vi "Execute_Row.vi"(3 "Simulate/Run":T2, 5 "Traverse line":T3 {"Row Duration (mins)" format="%#.1f"; "Row No" min=0; "Trace Gas Concentration (%)" min=0.0 format="%#.2f"; "Emission Rate (l/min)" format="%#.2f"; "Tunnel Speed" format="%#.2f"; "Start X" format="%#.2f"; "Start Y" format="%#.2f"; "Start Z" format="%#.2f"; "End X" format="%#.2f"; "End Y" format="%#.2f"; "End Z" format="%#.2f"; "Averaging time (min)" min=0.0 format="%#.2f"}) -> (1 "Status":T1, 2 "Traverse line out":T3 {"Row Duration (mins)" format="%#.1f"; "Row No" min=0; "Trace Gas Concentration (%)" min=0.0 format="%#.2f"; "Emission Rate (l/min)" format="%#.2f"; "Tunnel Speed" format="%#.2f"; "Start X" format="%#.2f"; "Start Y" format="%#.2f"; "Start Z" format="%#.2f"; "End X" format="%#.2f"; "End Y" format="%#.2f"; "End Z" format="%#.2f"; "Averaging time (min)" min=0.0 format="%#.2f"})   [LabVIEW 2014]
uses:
  Traverse_cluster.ctl
  Spacing.ctl
  Controls/Multi_run_mode.ctl
  Controls/User_Specific_mode.ctl
  Multi_Run_Status.ctl
  Controls/Setup.ctl
  Controls/Save_Data.ctl
  Globals/Constants_global.vi
  Globals/Extra_Commands_Global.vi
  Globals/Trav_pos_global.vi
panel:
  # "X           Y            Z"
  # "Start"
  # "End"
  # "X           Y            Z"
  # "Start"
  # "End"
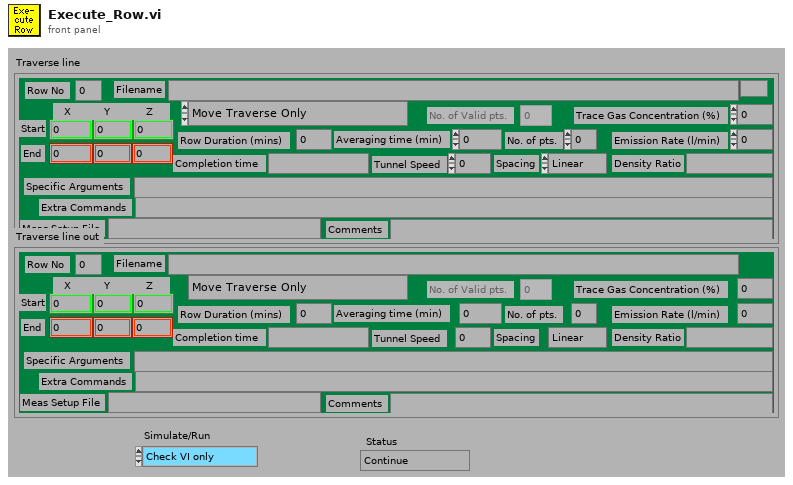
[diagram p1: front panel]
types:
  T1 = typedef "Multi_Run_Status.ctl" = enum16{"Continue", "Jump to Next Point", "Jump to Next Row", "Jump To Fall Back", "Terminate Run"}
  T2 = typedef "User_Specific_mode.ctl" = enum16{"Check VI only", "Run VI"}
  T3 = typedef "Traverse_cluster.ctl" = cluster{"Start X":dbl, "Start Y":dbl, "Start Z":dbl, "End X":dbl, "End Y":dbl, "End Z":dbl, "No. of pts.":i32, "Spacing":T4, "Filename":path, "Tunnel Speed":dbl, "Averaging time (min)":dbl, "Extra Commands":string, "Specific Arguments":string, "Emission Rate (l/min)":dbl, "Trace Gas Concentration (%)":dbl, "Density Ratio":string, "Comments":string, "Row No":i32, "Row Type Selector":T5, "Completion time":string, "Row Duration (mins)":dbl, "No. of Valid pts.":i32, "Meas Setup File":string}
  T4 = typedef "Spacing.ctl" = enum16{"Linear", "Log", "Gauss", "Specified", "N/A"}
  T5 = typedef "Multi_run_mode.ctl" = enum16{"Move Traverse Only", "Set Tunnel Speed Only", "Set Source Only", "Set Measurement Conditions", "Single Measurement", "Vertical Profile", "Lateral Profile", "Longitudinal Profile", "Explore Volume", "Multi-Axis Profile", "Auto Calibrate", "Meas Fast FID Bkgnd", "Check Beam Power", "Scanning Valve Measurement", "Run VI Named:", "Set ADAM Ch", "Wait (minutes)", "Send Message", "Synchronize With:", "Fall Back to this Row", "Turn Off Row Repeating", "Blank Row", "Traverse 3D Volume"}
  T6 = typedef "Save_Data.ctl" = enum16{"Save No Data", "Save Data"}
  T7 = typedef "Setup.ctl" = enum16{"Run Program", "Show Setup", "Save Current Setup", "Setup Front Panel"}
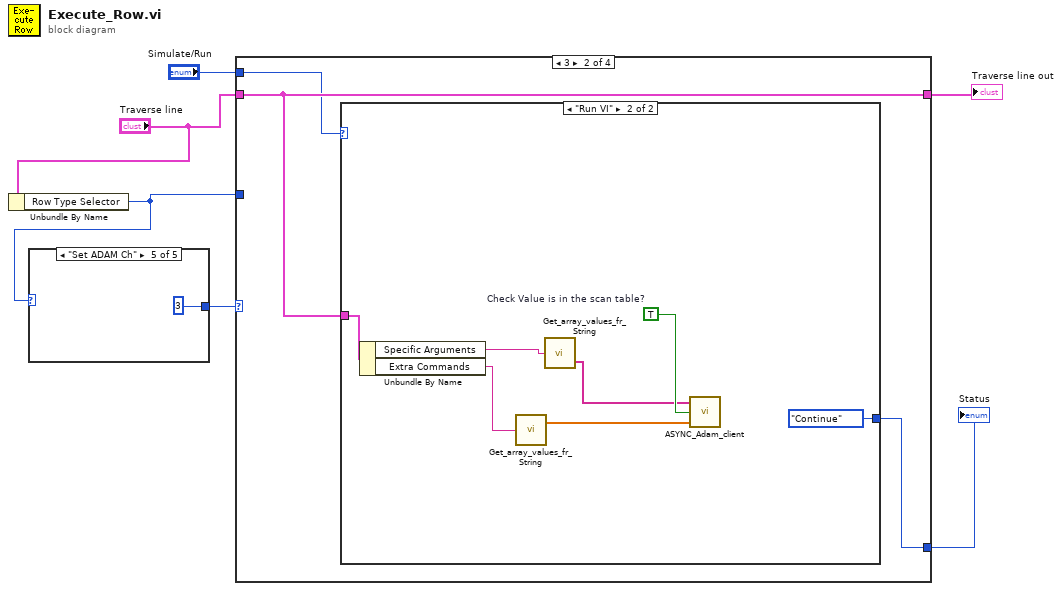
[diagram p0: block diagram]
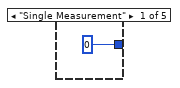
[diagram p2: hidden frame]
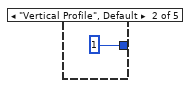
[diagram p3: hidden frame]
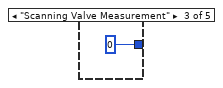
[diagram p4: hidden frame]
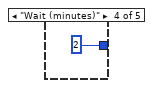
[diagram p5: hidden frame]
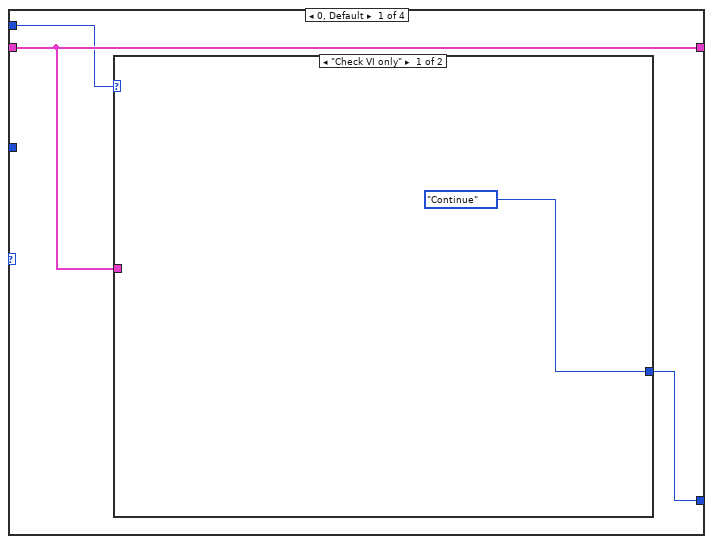
[diagram p6: hidden frame]
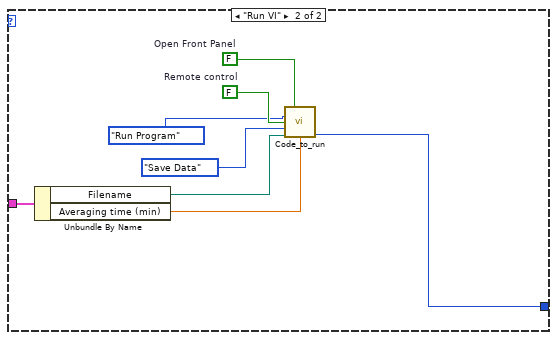
[diagram p7: hidden frame]
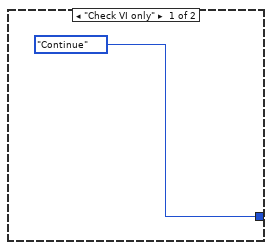
[diagram p8: hidden frame]
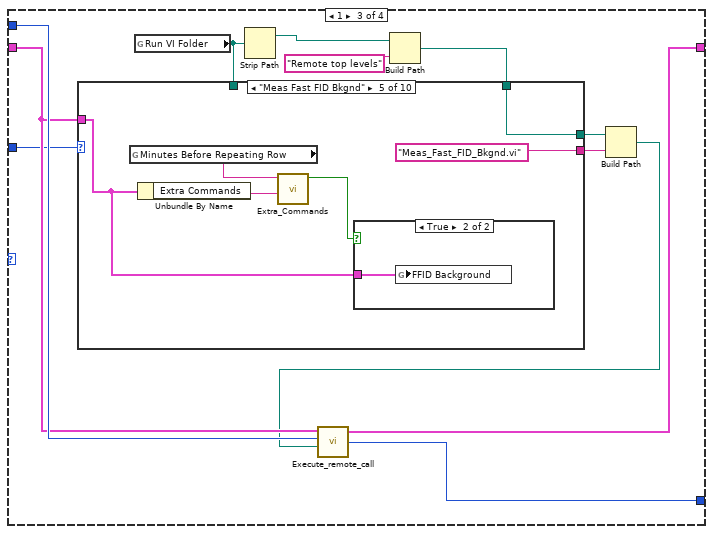
[diagram p9: hidden frame]
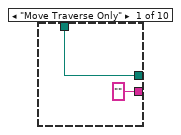
[diagram p10: hidden frame]
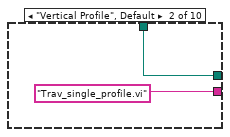
[diagram p11: hidden frame]
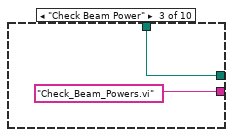
[diagram p12: hidden frame]
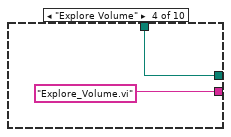
[diagram p13: hidden frame]
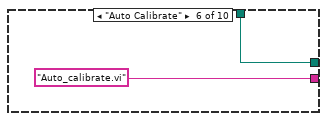
[diagram p15: hidden frame]
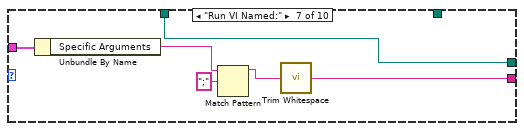
[diagram p16: hidden frame]
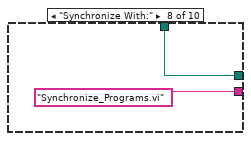
[diagram p17: hidden frame]
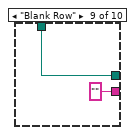
[diagram p18: hidden frame]
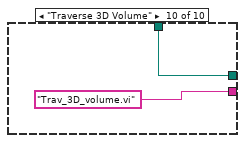
[diagram p19: hidden frame]
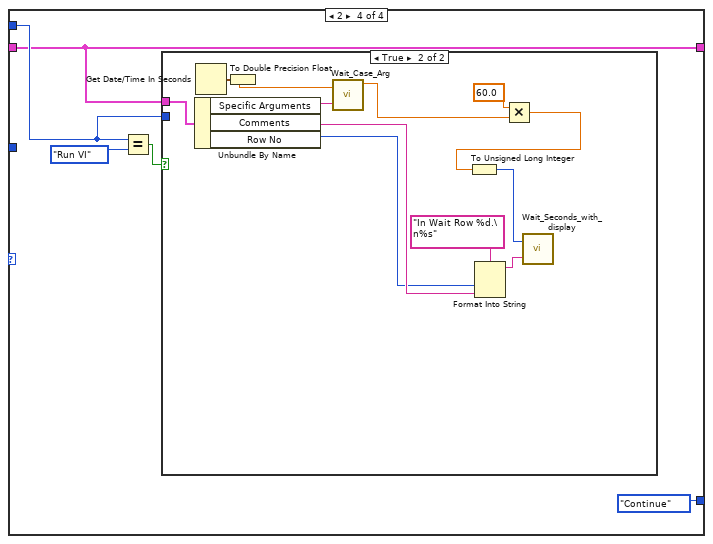
[diagram p20: hidden frame]
diagram:
  n1 = Unbundle By Name("Traverse line") -> ("Row Type Selector"=w2:T5)
  n2 = case shown="\"Set ADAM Ch\"" w2 {
    tunnel: [0 1 0 2 3] -> w3
    frame "Single Measurement" {
    }
    frame "Vertical Profile", Default {
    }
    frame "Scanning Valve Measurement" {
    }
    frame "Wait (minutes)" {
    }
    frame "Set ADAM Ch" {
    }
  }
  n3 = case shown="3" w3 {
    tunnel: [w14 w26 w42 Multi_Run_Status."Continue" ("Status")] -> w1
    tunnel: "Traverse line" -> [w13 w25 w44 w77]
    tunnel: [w13 w25 w46 w77] -> w6
    tunnel: "Simulate/Run" -> [w12 w24 w45 w79]
    tunnel: w2 -> [_ _ w43 _]
    frame 0, Default {
      n4 = case shown="\"Check VI only\"" w12 {
        tunnel: [Multi_Run_Status."Continue" ("Status") w23] -> w14
        tunnel: w13 -> [_ w22]
        frame "Check VI only" {
        }
        frame "Run VI" {
          w18 = FALSE  # Open Front Panel
          w20 = FALSE  # Remote control
          n5 = Unbundle By Name(w22) -> ("Filename"=w21:path, "Averaging time (min)"=w19:dbl)
          n6 = call "Code_to_run.vi"("Open Front Panel"=w18, "setup"=Setup."Run Program", "Remote control"=w20, "File"=Save_Data."Save Data", "Results Filename"=w21, "Averaging time (min)"=w19) -> ("Status"=w23:T1)  [unwired: 5 in, 4 out]
        }
      }
    }
    frame 3 {
      n7 = case shown="\"Run VI\"" w24 {
        tunnel: [Multi_Run_Status."Continue" ("Status") Multi_Run_Status."Continue" ("Status")] -> w26
        tunnel: w25 -> [_ w34]
        frame "Check VI only" {
        }
        frame "Run VI" {
          w32 = TRUE  # Check Value is in the scan table?
          n8 = Unbundle By Name(w34) -> ("Specific Arguments"=w31:string, "Extra Commands"=w29:string)
          n9 = call "Get_array_values_fr_String.vi"("String Value"=w29) -> ("Numeric Array"=w28:dbl[])  [unwired: 1 out]
          n10 = call "Get_array_values_fr_String.vi"("String Value"=w31) -> ("String array"=w30:string[])  [unwired: 1 out]
          n11 = call "ASYNC_Adam_client.vi"("Values"=w28, "Check Value is in the scan table?"=w32, "Channel Names"=w30) -> ()  [unwired: 2 out]
        }
      }
    }
    frame 1 {
      n12 = global read "Constants_global.vi" "Run VI Folder"() -> (w35:path)
      n13 = Strip Path(path=w35) -> (stripped path=w36:path)  [unwired: 1 out]
      n14 = Build Path(base path=w36, name or relative path="Remote top levels") -> (appended path=w40:path)
      n15 = case shown="\"Meas Fast FID Bkgnd\"" w43 {
        tunnel: w40 -> [w48 w50 w52 w54 w60 w63 _ w71 w73 w75]
        tunnel: w44 -> [_ _ _ _ w55 _ w69 _ _ _]
        tunnel: [w48 w50 w52 w54 w60 w63 w68 w71 w73 w75] -> w39
        tunnel: ["" ("name") "Trav_single_profile.vi" "Check_Beam_Powers.vi" "Explore_Volume.vi" "Meas_Fast_FID_Bkgnd.vi" "Auto_calibrate.vi" w64 "Synchronize_Programs.vi" "" ("name") "Trav_3D_volume.vi" ("name")] -> w38
        tunnel: w35 -> [_ _ _ _ _ _ w68 _ _ _]
        frame "Move Traverse Only" {
        }
        frame "Vertical Profile", Default {
        }
        frame "Check Beam Power" {
        }
        frame "Explore Volume" {
        }
        frame "Meas Fast FID Bkgnd" {
          n16 = global read "Extra_Commands_Global.vi" "Minutes Before Repeating Row"() -> (w58:string)
          n17 = Unbundle By Name(w55) -> ("Extra Commands"=w57:string)
          n18 = call "Extra_Commands.vi"("String to Search"=w57, "Command"=w58) -> ("Command Found"=w56:bool)  [unwired: 1 in, 4 out]
          n19 = case shown="True" w56 {
            tunnel: w55 -> [_ w61]
            frame False {
            }
            frame True {
              n20 = global write "Trav_pos_global.vi" "FFID Background"(w61) -> ()
            }
          }
        }
        frame "Auto Calibrate" {
        }
        frame "Run VI Named:" {
          n21 = Unbundle By Name(w69) -> ("Specific Arguments"=w66:string)
          n22 = Match Pattern(string=w66, regular expression=";") -> (before substring=w65:string)  [unwired: 4 out]
          n23 = call <vilib>:"Trim Whitespace.vi"("string"=w65) -> ("trimmed string"=w64:string)  [unwired: 1 in]
        }
        frame "Synchronize With:" {
        }
        frame "Blank Row" {
        }
        frame "Traverse 3D Volume" {
        }
      }
      n24 = Build Path(base path=w39, name or relative path=w38) -> (appended path=w37:path)
      n25 = call "Execute_remote_call.vi"("Traverse line"=w44, "Simulate/Run"=w45, "VI to run"=w37) -> ("Traverse Out"=w46:T3, "Status"=w42:T1)  [unwired: 1 in, 3 out]
    }
    frame 2 {
      n26 = Equal?(x=w79, y=User_Specific_mode."Run VI" ("Simulate/Run")) -> (x = y?=w78:bool)
      n27 = case shown="True" w78 {
        tunnel: w77 -> [_ w86]
        tunnel: w79 -> [_ _]
        frame False {
        }
        frame True {
          n28 = Unbundle By Name(w86) -> ("Specific Arguments"=w87:string, "Comments"=w82:string, "Row No"=w81:i32)
          n29 = Get Date/Time In Seconds() -> (seconds since 1Jan1904=w85:timestamp)
          n30 = To Double Precision Float(number=w85) -> (double precision float=w88:dbl)
          n31 = call "Wait_Case_Arg.vi"("Specific Argument"=w87, "seconds since 1Jan1904"=w88) -> ("Minutes To Wait"=w89:dbl)  [unwired: 4 out]
          n32 = Format Into String(format string="In Wait Row %d.\n%s", w81, w82) -> (resulting string=w84:string)  [unwired: 2 in, 1 out]
          n33 = Multiply(x=60.0, y=w89) -> (x*y=w90:dbl)
          n34 = To Unsigned Long Integer(number=w90) -> (unsigned 32bit integer=w91:u32)
          n35 = call "Wait_Seconds_with_display.vi"("Message"=w84, "Seconds to wait"=w91) -> ()  [unwired: 2 out]
        }
      }
    }
  }
  "Traverse line out" <- w6
  "Status" <- w1
